vi "GetDiagramOutputs.vi"(6 "error in":errorcluster, 9 "FlatSequenceFrame in":refnum<class "FlatSequenceFrame.lvclass">) -> (0 "error out":errorcluster, 3 "FlatSequenceFrame out":refnum<class "FlatSequenceFrame.lvclass">, 4 "output terminals":refnum<class "Terminal.lvclass">[][](array[class]))   [LabVIEW 2014, in "FlatSequenceFrame.lvclass"]
uses:
  FlatSequenceFrame.lvclass
  Terminal/Terminal.lvclass
  FlatSequenceFrame.lvclass/FlatSequenceFrame.ctl
  FlatSequenceInnerTunnel/FlatSequenceInnerTunnel.lvclass/FlatSequenceInnerTunnel.ctl
  FlatSequenceOuterTunnel/FlatSequenceOuterTunnel.lvclass/FlatSequenceOuterTunnel.ctl
  FlatSequenceInnerTunnel/FlatSequenceInnerTunnel.lvclass
  FlatSequenceOuterTunnel/FlatSequenceOuterTunnel.lvclass
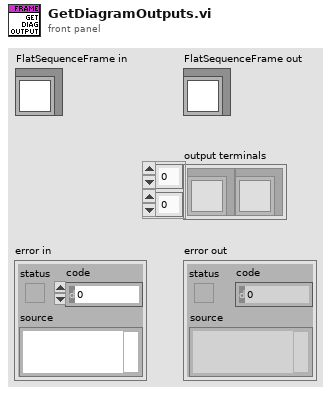
[diagram p1: front panel]
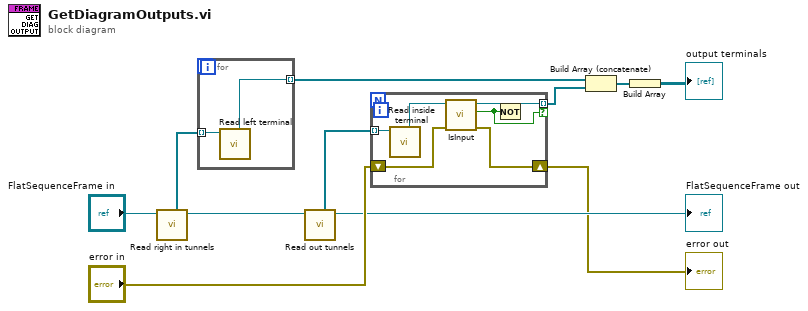
[diagram p0: block diagram]
diagram:
  n1 = call "Read right in tunnels.vi"("FlatSequenceFrame in"="FlatSequenceFrame in") -> ("FlatSequenceFrame out"=w10:refnum<class "FlatSequenceFrame.lvclass">, "right in tunnels"=w11:refnum<class "FlatSequenceInnerTunnel.lvclass">[])  [unwired: 7 in]
  n2 = for {
    tunnel: w11 -> [w13] mode=indexing
    tunnel: [w12] -> w8 mode=indexing
    n3 = call "Read left terminal.vi"("FlatSequenceInnerTunnel in"=w13) -> ("left terminal"=w12:refnum<class "Terminal.lvclass">)  [unwired: 7 in, 1 out]
  }
  n4 = call "Read out tunnels.vi"("FlatSequenceFrame in"=w10) -> ("FlatSequenceFrame out"=→"FlatSequenceFrame out":refnum<class "FlatSequenceFrame.lvclass">, "out tunnels"=w9:refnum<class "FlatSequenceOuterTunnel.lvclass">[])  [unwired: 7 in]
  n5 = for {
    tunnel: w9 -> [w19] mode=indexing
    tunnel: [w17] -> w7 mode=indexing if=w14
    shift-right: [w15] -> w2
    shift-left: "error in" -> [w16]
    n6 = call "Read inside terminal.vi"("FlatSequenceInnerTunnel in"=w19) -> ("inside terminal"=w18:refnum<class "Terminal.lvclass">)  [unwired: 7 in, 1 out]
    n7 = call-dynamic "IsInput.vi"("error in"=w16, "Terminal in"=w18) -> ("error out"=w15:errorcluster, "input"=w14:bool, "Terminal out"=w17:refnum<class "Terminal.lvclass">)  [unwired: 5 in]
    n8 = Not(x=w14) -> ()  [unwired: 1 out]
  }
  "error out" <- w2
  n9 = Build Array (concatenate)(w8, w7) -> (w6:refnum<class "Terminal.lvclass">[])
  n10 = Build Array(w6) -> (→"output terminals":refnum<class "Terminal.lvclass">[][])
